vi "Read Number of Dims.vi"(9 "Array in":refnum<class "Array.lvclass">) -> (3 "Array out":refnum<class "Array.lvclass">, 4 "Number of Dims":u32)   [LabVIEW 2014, in "Array.lvclass"]
uses:
  Array.lvclass
  Array.lvclass/Array.ctl
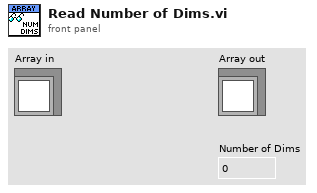
[diagram p1: front panel]
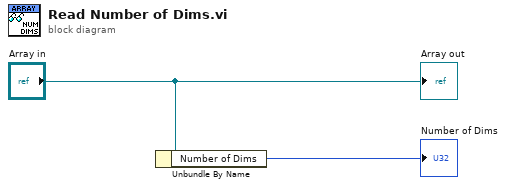
[diagram p0: block diagram]
diagram:
  n1 = Unbundle By Name("Array in") -> ("Number of Dims"=→"Number of Dims":u32)
  "Array out" <- "Array in"
